vi "Log Temperature.vi"(8 "error in":errorcluster, 9 "LogData":bool, 11 "Data in":T1 {"LogStartTime" format="%<%x %.3X>T"}) -> (0 "error out":errorcluster, 1 "New Measure?":bool, 3 "Data Out":T1 {"LogStartTime" format="%<%x %.3X>T"})   [LabVIEW 2023]
uses:
  controls/UI Data.ctl
  <vilib>/NI/Modbus Library/API/Master/Modbus Master.lvclass
  LibreVNA/LibreVNA.lvclass
  <vilib>/Utility/file.llb/Write Delimited Spreadsheet (DBL).vi
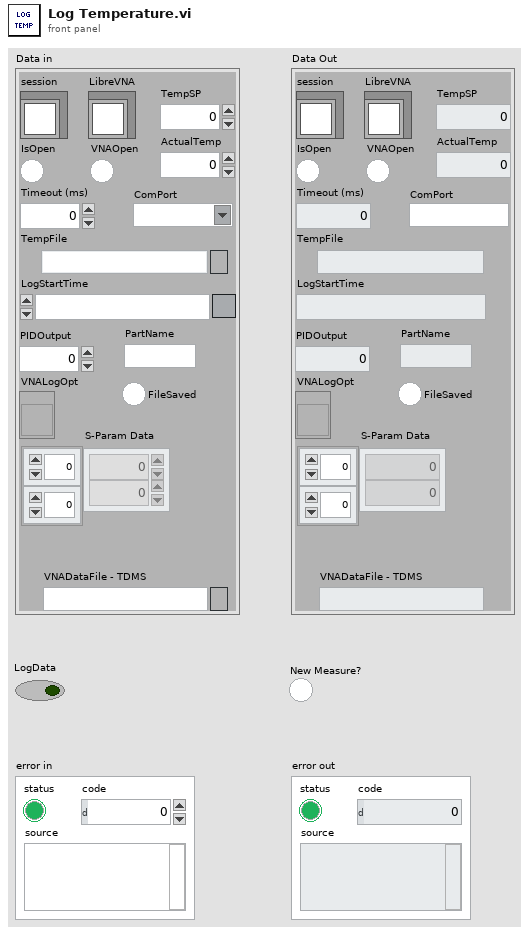
[diagram p1: front panel]
types:
  T1 = typedef "UI Data.ctl" = cluster{"session":refnum<class "Modbus Master.lvclass">, "IsOpen":bool, "Timeout (ms)":i32, "TempFile":path, "LogStartTime":timestamp, "LibreVNA":refnum<class "LibreVNA.lvclass">, "VNAOpen":bool, "TempSP":dbl, "ActualTemp":dbl, "FileSaved":bool, "PIDOutput":dbl, "VNALogOpt":refnum<vi>, "PartName":string, "ComPort":refnum<visa-resource-name>, "S-Param Data":dbl[][], "VNADataFile - TDMS":path}
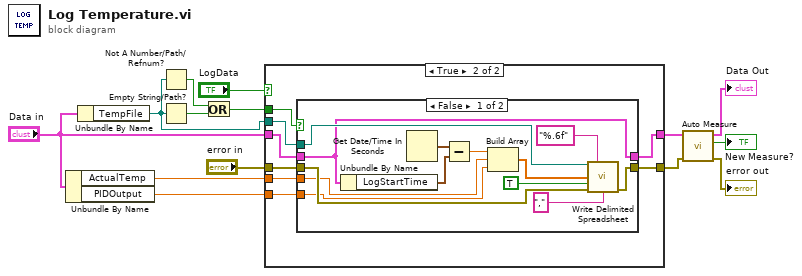
[diagram p0: block diagram]
diagram:
  n1 = Unbundle By Name("Data in") -> ("ActualTemp"=w3:dbl, "PIDOutput"=w4:dbl)
  n2 = Unbundle By Name("Data in") -> ("TempFile"=w9:path)
  n3 = Not A Number/Path/Refnum?(number/path/refnum=w9) -> (NaN/Path/Refnum?=w12:bool)
  n4 = Empty String/Path?(string/path=w9) -> (empty?=w11:bool)
  n5 = Or(x=w12, y=w11) -> (x .or. y?=w10:bool)
  n6 = case shown="True" "LogData" {
    tunnel: w9 -> [_ w24]
    tunnel: [w16 w22] -> w8
    tunnel: "Data in" -> [w16 w23]
    tunnel: "error in" -> [w15 w21]
    tunnel: [w15 w20] -> w2
    tunnel: w10 -> [_ w19]
    tunnel: w3 -> [_ w18]
    tunnel: w4 -> [_ w17]
    frame False {
    }
    frame True {
      n7 = case shown="False" w19 {
        tunnel: w24 -> [w37 _]
        tunnel: w23 -> [w32 w38]
        tunnel: [w32 w38] -> w22
        tunnel: w21 -> [w34 w39]
        tunnel: [w33 w39] -> w20
        tunnel: w18 -> [w28 _]
        tunnel: w17 -> [w25 _]
        frame False {
          n8 = Unbundle By Name(w32) -> ("LogStartTime"=w31:timestamp)
          n9 = Get Date/Time In Seconds() -> (seconds since 1Jan1904=w30:timestamp)
          n10 = Subtract(x=w30, y=w31) -> (x-y=w29:dbl)
          n11 = Build Array(w29, w28, w25) -> (w27:dbl[])
          n12 = call-poly <vilib>:"Write Delimited Spreadsheet.vi"("file path (dialog if empty)"=w37, "format (%.3f)"="%.6f" ("format (%s)"), "1D data"=w27, "append to file? (new file:F)"=TRUE, "error in (no error)"=w34, "delimiter (\\t)"="," ("delimiter (\\t)")) -> ("error out"=w33:errorcluster)  [unwired: 8 in, 1 out]
        }
        frame True {
        }
      }
    }
  }
  n13 = call "Auto Measure.vi"("error in"=w2, "Data in"=w8) -> ("error out"=→"error out":errorcluster, "New Measure?"=→"New Measure?":bool, "Data Out"=→"Data Out":T1)  [unwired: 3 in]
